vi "TCP Send Image.vi"(0 "Connection ID":refnum<k5>, 7 "Image Stack (U16)":u16[][][](array[numeric]), 11 "Error In":errorcluster) -> (4 "Connection ID Out":refnum<k5>, 8 "Success?":bool, 15 "Error Out":errorcluster)   [LabVIEW 2016]
panel:
  out "Image Size":i32[](array[numeric])
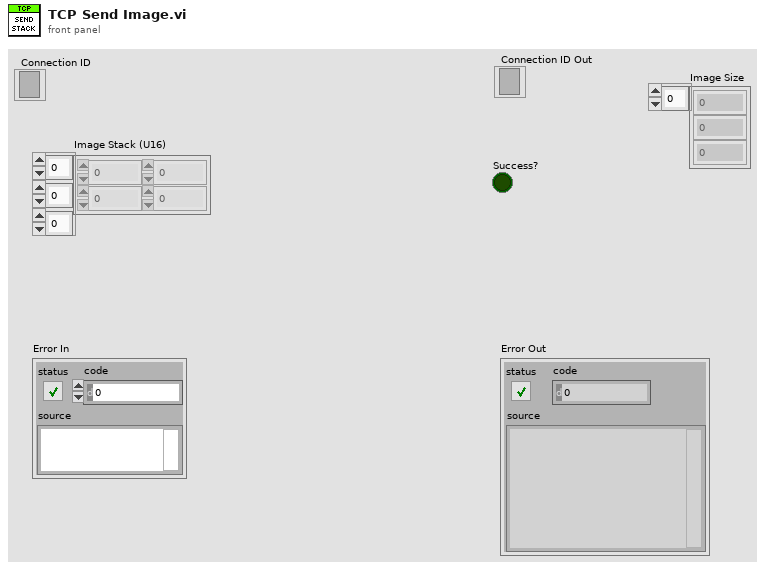
[diagram p1: front panel]
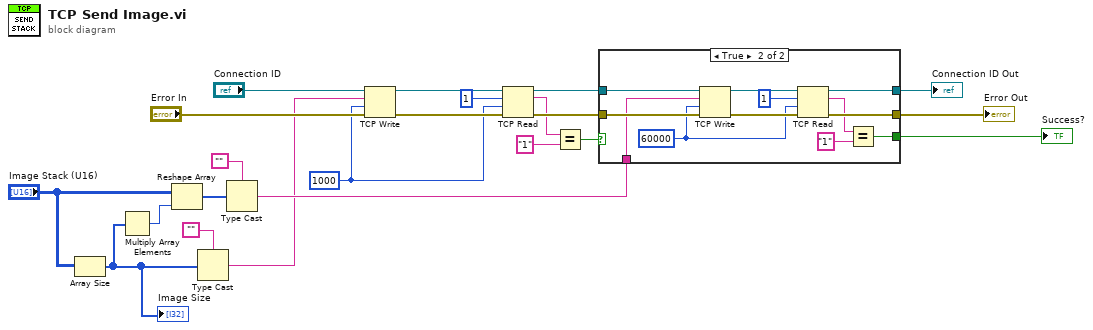
[diagram p0: block diagram]
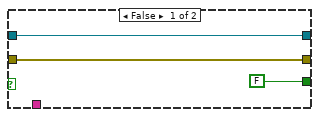
[diagram p2: hidden frame]
diagram:
  w4 = 1000 ("timeout ms (25000)")
  n1 = Array Size(array="Image Stack (U16)") -> (size(s)=w2:i32[])
  "Image Size" <- w2
  n2 = Multiply Array Elements(1:w2) -> (0:w14:i32)
  n3 = Reshape Array("Image Stack (U16)", w14) -> (w21:u16[])
  n4 = Type Cast(type="", x=w2) -> (*(type *) &x=w1:string)
  n5 = Type Cast(type="", x=w21) -> (*(type *) &x=w5:string)
  n6 = TCP Write(connection ID="Connection ID", data in=w1, error in (no error)="Error In", 9:w4) -> (connection ID out=w18:refnum<k5>, error out=w12:errorcluster)  [unwired: 1 out]
  n7 = TCP Read(connection ID=w18, bytes to read=1, error in (no error)=w12, 9:w4) -> (connection ID out=w17:refnum<k5>, data out=w7:string, error out=w11:errorcluster)  [unwired: 1 in]
  n8 = Equal?(x=w7, y="1") -> (x = y?=w6:bool)
  n9 = case shown="True" w6 {
    tunnel: w17 -> [w25 w37]
    tunnel: [w25 w35] -> w16
    tunnel: w11 -> [w24 w34]
    tunnel: [w24 w32] -> w10
    tunnel: w5 -> [_ w31]
    tunnel: [FALSE w27] -> w3
    frame False {
    }
    frame True {
      w26 = 60000 ("timeout ms (25000)")
      n10 = TCP Write(connection ID=w37, data in=w31, error in (no error)=w34, 9:w26) -> (connection ID out=w36:refnum<k5>, error out=w33:errorcluster)  [unwired: 1 out]
      n11 = TCP Read(connection ID=w36, bytes to read=1, error in (no error)=w33, 9:w26) -> (connection ID out=w35:refnum<k5>, data out=w28:string, error out=w32:errorcluster)  [unwired: 1 in]
      n12 = Equal?(x=w28, y="1") -> (x = y?=w27:bool)
    }
  }
  "Connection ID Out" <- w16
  "Error Out" <- w10
  "Success?" <- w3
